vi "Parse_Flow_Arguments.vi"(2 "Flow Command String":string="Flow", 3 "Argument List":string[](array[string])) -> (0 "Flow Array":dbl[](array[numeric]), 1 "New Argument List":string[](array[string]))   [LabVIEW 2011]
doc: "This VI parses an argument list that contains flow arguments and values. The reason this is necessary is because the growth sequence editor code does not store flow values as strings in the argument list, but rather as numerical double values in a separate array designated the \"Flow Array\". This VI will remove the \"Flow\" arguments in the argument list and convert them to numerical double values where they will be returned in the \"Flow Array\" output."
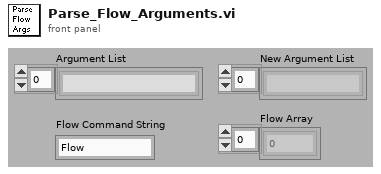
[diagram p1: front panel]
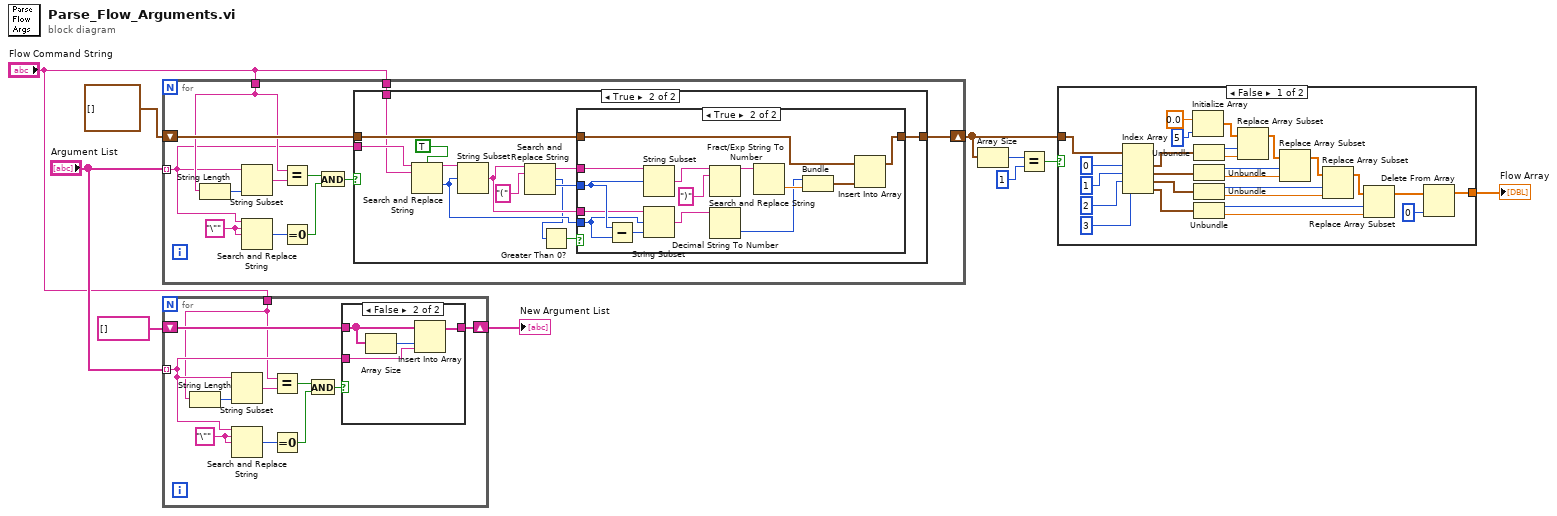
[diagram p0: block diagram]
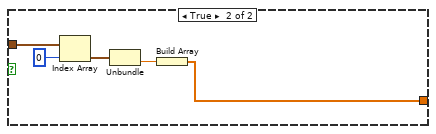
[diagram p2: hidden frame]
diagram:
  n1 = for {
    tunnel: "Argument List" -> [w16] mode=indexing
    shift-right: [w22] -> w4
    shift-left: cluster{"offset past number":i32, dbl}[] [] -> [w21]
    tunnel: "Flow Command String" -> [w20]
    tunnel: "Flow Command String" -> [w18]
    w15 = "\"" ("search string")
    n2 = String Length(string=w18) -> (length=w19:i32)
    n3 = String Subset(string=w16, length (rest)=w19) -> (substring=w17:string)  [unwired: 1 out]
    n4 = Search and Replace String(input string=w16, search string=w15, replace string=w15) -> (number of replacements=w14:i32)  [unwired: 1 in, 7 out]
    n5 = Equal?(x=w18, y=w17) -> (x = y?=w12:bool)
    n6 = Equal To 0?(x=w14) -> (x = 0?=w11:bool)
    n7 = And(x=w12, y=w11) -> (x .and. y?=w13:bool)
    n8 = case shown="True" w13 {
      tunnel: w16 -> [_ w35]
      tunnel: [w23 w28] -> w22
      tunnel: w21 -> [w23 w29]
      tunnel: w20 -> [_ w24]
      frame False {
      }
      frame True {
        n9 = Search and Replace String(case sensitive?=TRUE ("ignore case? (F)"), input string=w35, search string=w24) -> (result string=w34:string, offset past replacement=w31:i32)  [unwired: 1 in, 6 out]
        n10 = String Subset(string=w34, offset (0)=w31) -> (substring=w30:string)  [unwired: 1 out]
        n11 = Search and Replace String(input string=w30, search string="(") -> (result string=w33:string, number of replacements=w26:i32, offset past replacement=w32:i32)  [unwired: 1 in, 6 out]
        n12 = Greater Than 0?(x=w26) -> (x > 0?=w27:bool)
        n13 = case shown="True" w27 {
          tunnel: w33 -> [_ w49]
          tunnel: w32 -> [_ w47]
          tunnel: w31 -> [_ w46]
          tunnel: w30 -> [_ w45]
          tunnel: w29 -> [w37 w40]
          tunnel: [w37 w39] -> w28
          frame False {
          }
          frame True {
            n14 = Subtract(x=w47, y=w46) -> (x-y=w48:i32)
            n15 = String Subset(string=w49, offset (0)=w47) -> (substring=w51:string)  [unwired: 1 out]
            n16 = String Subset(string=w45, offset (0)=w46, length (rest)=w48) -> (substring=w44:string)
            n17 = Search and Replace String(input string=w51, search string=")" ("replace string (\"\")")) -> (result string=w43:string)  [unwired: 1 in, 8 out]
            n18 = Decimal String To Number(string=w44) -> (number=w38:i32)  [unwired: 3 out]
            n19 = Fract/Exp String To Number(string=w43) -> (number=w42:dbl)  [unwired: 4 out]
            n20 = Bundle(w38, w42) -> (w41:cluster{i32, dbl})  [unwired: 1 out]
            n21 = Insert Into Array(array=w40, new element=w41) -> (w39:cluster{"offset past number":i32, dbl}[])  [unwired: 1 in]
          }
        }
      }
    }
  }
  n22 = for {
    tunnel: "Argument List" -> [w53] mode=indexing
    shift-right: [w61] -> w6
    shift-left: string[] [] -> [w62]
    tunnel: "Flow Command String" -> [w52]
    w57 = "\"" ("search string")
    n23 = String Length(string=w52) -> (length=w55:i32)
    n24 = String Subset(string=w53, length (rest)=w55) -> (substring=w56:string)  [unwired: 1 out]
    n25 = Search and Replace String(input string=w53, search string=w57, replace string=w57) -> (number of replacements=w58:i32)  [unwired: 1 in, 7 out]
    n26 = Equal?(x=w52, y=w56) -> (x = y?=w59:bool)
    n27 = Equal To 0?(x=w58) -> (x = 0?=w60:bool)
    n28 = And(x=w59, y=w60) -> (x .and. y?=w54:bool)
    n29 = case shown="False" w54 {
      tunnel: w53 -> [_ w67]
      tunnel: w62 -> [w63 w65]
      tunnel: [w63 w64] -> w61
      frame True {
      }
      frame False {
        n30 = Array Size(array=w65) -> (size(s)=w66:i32)
        n31 = Insert Into Array(array=w65, index=w66, new element=w67) -> (w64:string[])
      }
    }
  }
  "New Argument List" <- w6
  n32 = Array Size(array=w4) -> (size(s)=w3:i32)
  n33 = Equal?(x=w3, y=1) -> (x = y?=w1:bool)
  n34 = case shown="False" w1 {
    tunnel: w4 -> [w84 w98]
    tunnel: [w70 w94] -> w9
    frame False {
      n35 = Index Array(array=w84, index #1=0 ("index"), index #2=1 ("index"), index #3=2 ("index"), index #4=3 ("index")) -> (element #1=w89:cluster{"offset past number":i32, dbl}, element #2=w88:cluster{"offset past number":i32, dbl}, element #3=w87:cluster{"offset past number":i32, dbl}, element #4=w86:cluster{"offset past number":i32, dbl})
      n36 = Initialize Array(0.0 ("element"), 5 ("dimension size")) -> (w82:dbl[])
      n37 = Unbundle(w89) -> ("offset past number"=w81:i32, w80:dbl)
      n38 = Unbundle(w88) -> ("offset past number"=w79:i32, w78:dbl)
      n39 = Unbundle(w87) -> ("offset past number"=w76:i32, w75:dbl)
      n40 = Unbundle(w86) -> ("offset past number"=w72:i32, w71:dbl)
      n41 = Replace Array Subset(array=w82, new element=w80, index=w81) -> (w77:dbl[])
      n42 = Replace Array Subset(array=w77, new element=w78, index=w79) -> (w74:dbl[])
      n43 = Replace Array Subset(array=w74, new element=w75, index=w76) -> (w73:dbl[])
      n44 = Replace Array Subset(array=w73, new element=w71, index=w72) -> (w68:dbl[])
      n45 = Delete From Array(array=w68, index=0) -> (array with subset deleted=w70:dbl[])  [unwired: 1 in, 1 out]
    }
    frame True {
      n46 = Index Array(array=w98, index=0) -> (element=w96:cluster{"offset past number":i32, dbl})
      n47 = Unbundle(w96) -> (w95:dbl)  [unwired: 1 out]
      n48 = Build Array(w95) -> (w94:dbl[])
    }
  }
  "Flow Array" <- w9
